vi "Char to U8.vi"(1 "Char":string) -> (0 "U8":u8)   [LabVIEW 2020]
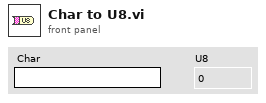
[diagram p1: front panel]
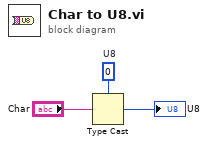
[diagram p0: block diagram]
diagram:
  w2 = u8 0  # U8
  n1 = Type Cast(type=w2, x="Char") -> (*(type *) &x=→"U8":u8)
